vi "create.ReduceSizeBase.vi"(8 "error in (no error)":errorcluster, 11 "ReduceSizeBase in":refnum<class "ReduceSizeBase.lvclass">) -> (0 "error out":errorcluster, 3 "ReduceSizeBase out":refnum<class "ReduceSizeBase.lvclass">)   [LabVIEW 2020, in "ReduceSizeBase.lvclass"]
uses:
  ReduceSizeBase.lvclass
  FieldSpec.ctl
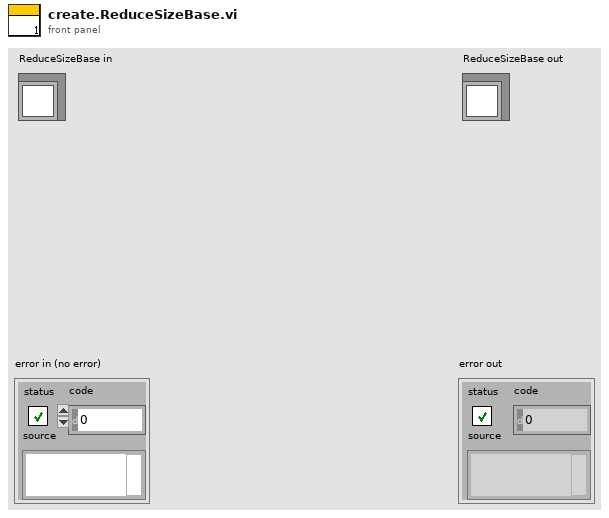
[diagram p1: front panel]
types:
  T1 = typedef "FieldSpec.ctl" = cluster{"Name":string, "Offset":i32, "Length":i32, "FieldType":enum16{"Alphanumeric", "Binary", "BinaryLongPrice", "BinaryShortPrice", "BitField", "PrintableAscii", "Value"}, "FieldValue":variant}
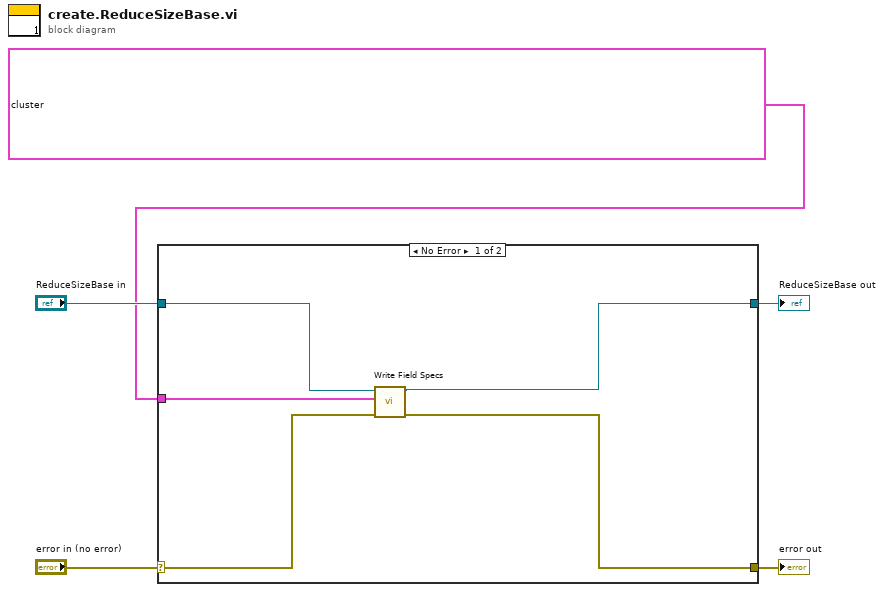
[diagram p0: block diagram]
diagram:
  n1 = case shown="No Error" "error in (no error)" {
    selector: "error in (no error)" -> [w9 w12]
    tunnel: [w8 w12] -> w4
    tunnel: [w7 w11] -> w2
    tunnel: "ReduceSizeBase in" -> [w6 w11]
    tunnel: T1[] [{"Name"="Length", "Offset"=0, "Length"=1, "FieldType"=enum."Binary", "FieldValue"=variant}, {"Name"="MessageType", "Offset"=1, "Length"=1, "FieldType"=enum."Value", "FieldValue"=variant}, {"Name"="Time Offset", "Offset"=2, "Length"=4, "FieldType"=enum."Binary", "FieldValue"=variant}, {"Name"="Order Id", "Offset"=6, "Length"=8, "FieldType"=enum."Binary", "FieldValue"=variant}, {"Name"="Canceled Quantity", "Offset"=14, "Length"=4, "FieldType"=enum."Binary", "FieldValue"=variant}] ("appended array") -> [w10 _]
    frame No Error {
      n2 = call-dynamic "Write Field Specs.vi"("error in (no error)"=w9, "Field Specs"=w10, "MessageBase in"=w6) -> ("error out"=w8:errorcluster, "MessageBase out"=w7:refnum<class "ReduceSizeBase.lvclass">)  [unwired: 7 in]
    }
    frame Error {
    }
  }
  "error out" <- w4
  "ReduceSizeBase out" <- w2
